vi "niFPGA I32xI32 Dot Product - 3 elements MSB.vi"(0 "A[]":i32[](array[numeric])=[0, 0, 0], 5 "B[]":i32[](array[numeric])=[0, 0, 0]) -> (7 "A.B [Hi I32]":i32=2838 format="%08x")   [LabVIEW 2017]
uses:
  <vilib>/Platform/TimedLoop/XDataNode/timing_clust.ctl
  <vilib>/Platform/TimedLoop/XDataNode/nitl_modes.ctl
  <vilib>/Platform/TimedLoop/XDataNode/wakeup.ctl
  <vilib>/Platform/TimedLoop/XDataNode/XDataNode.xnode
  <vilib>/Platform/TimedLoop/XDataNode/XDNodeRunTimeDep.lvlib
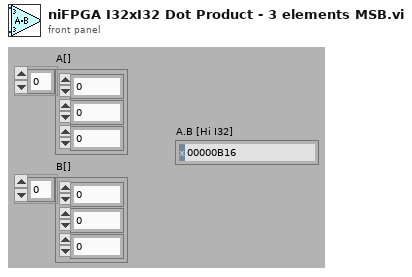
[diagram p1: front panel]
types:
  T1 = typedef "XDNodeRunTimeDep.lvlib/timing_clust.ctl" = cluster{"Expected End [f-1]":u64, "Actual End [f-1]":u64, "Finished Late? [f-1]":bool, "Expected End [i-1]":u64, "Actual End [i-1]":u64, "Finished Late? [i-1]":bool, "Expected Start [i]":u64, "Actual Start [i]":u64, "Expected Start [f]":u64, "Actual Start [f]":u64, "Source Name":string, "Structure Name":string, "Period":i64, "Deadline":i64, "Offset":i64, "Start":i64, "Priority":i32, "Timeout":i32, "Mode":T2, "Wakeup Reason":T3, "Error":errorcluster, "Source Type":string, "Secondary Source Type":string, "Global End Time":u64, "Global Start Time":u64, "Frame Duration":u64, "Iteration Duration":u64, "Assigned CPU":i32, "I/O Scan Engine Mode":u32}
  T2 = typedef "XDNodeRunTimeDep.lvlib/nitl_modes.ctl" = enum32{"No Change", "Process missed periods, maintain original phase", "Discard missed periods, maintain original phase", "Process missed periods, ignore original phase", "Discard missed periods, ignore original phase"}
  T3 = typedef "XDNodeRunTimeDep.lvlib/wakeup.ctl" = enum32{"Normal", "Aborted", "Asynchronous wakeup", "Timing source error", "Timed loop error", "Timeout"}
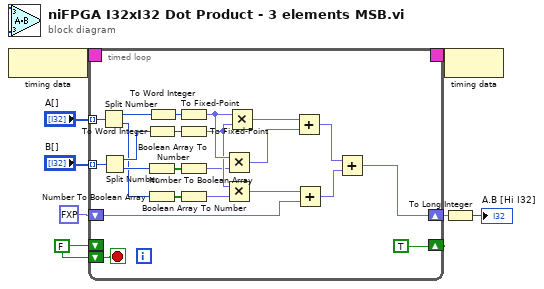
[diagram p0: block diagram]
diagram:
  w4 = FALSE
  n1 = node-c288() -> (w8:T1)
  n2 = timed-loop {
    shift-left: w4 -> [_]
    shift-right: [TRUE] -> _
    shift-left: fxp<+/-,32,32> 0.0 -> [w10]
    shift-right: [w9] -> w2
    tunnel: "A[]" -> [w12] mode=indexing
    tunnel: "B[]" -> [w11] mode=indexing
    timing: w8 -> [_]
    timing-out: [_] -> w7
    shift-left: w4 -> [w30]
    stop <- w30 stop-if-true
    n3 = Split Number(x=w12) -> (hi(x)=w28:u16, lo(x)=w14:u16)
    n4 = Split Number(x=w11) -> (hi(x)=w29:u16, lo(x)=w17:u16)
    n5 = To Word Integer(number=w29) -> (16bit integer=w25:i16)
    n6 = Number To Boolean Array(number=w17) -> (Boolean array=w18:bool[])
    n7 = Number To Boolean Array(number=w14) -> (Boolean array=w15:bool[])
    n8 = To Word Integer(number=w28) -> (16bit integer=w27:i16)
    n9 = To Fixed-Point(number=w27) -> (fixed-point=w26:fxp<+/-,16,16>)  [unwired: 1 out]
    n10 = To Fixed-Point(number=w25) -> (fixed-point=w24:fxp<+/-,16,16>)  [unwired: 1 out]
    n11 = Boolean Array To Number(Boolean array=w18) -> (number=w16:fxp<+,16,0>)
    n12 = Boolean Array To Number(Boolean array=w15) -> (number=w13:fxp<+,16,0>)
    n13 = Multiply(x=w26, y=w16) -> (x*y=w22:fxp<+/-,16,16>)
    n14 = Multiply(x=w24, y=w13) -> (x*y=w21:fxp<+/-,16,16>)
    n15 = Multiply(x=w26, y=w24) -> (x*y=w23:fxp<+/-,32,32>)
    n16 = Add(x=w23, y=w22) -> (x+y=w20:fxp<+/-,32,32>)
    n17 = Add(x=w21, y=w10) -> (x+y=w19:fxp<+/-,33,33>)
    n18 = Add(x=w20, y=w19) -> (x+y=w9:fxp<+/-,32,32>)
  }
  n19 = node-c288(w7) -> ()
  n20 = To Long Integer(number=w2) -> (32bit integer=→"A.B [Hi I32]":i32)
